vi "Write Wheel Speed Global.vi"(0 "Wheel 4":dbl, 1 "Wheel 3":dbl, 2 "Wheel 2":dbl, 3 "Wheel 1":dbl) -> ()   [LabVIEW 2016]
uses:
  Main/Robot Global Data.vi
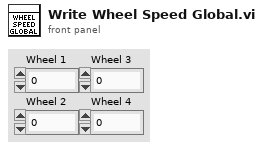
[diagram p1: front panel]
types:
  T1 = cluster{"Wheel 1":dbl, "Wheel 2":dbl, "Wheel 3":dbl, "Wheel 4":dbl}
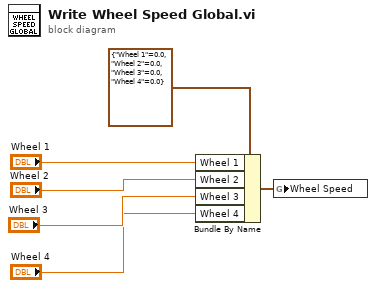
[diagram p0: block diagram]
diagram:
  n1 = Bundle By Name(cluster=T1 {"Wheel 1"=0.0, "Wheel 2"=0.0, "Wheel 3"=0.0, "Wheel 4"=0.0} ("input cluster"), "Wheel 1"="Wheel 1", "Wheel 2"="Wheel 2", "Wheel 3"="Wheel 3", "Wheel 4"="Wheel 4") -> (w5:T1)
  n2 = global write "Robot Global Data.vi" "Wheel Speed"(w5) -> ()
